vi "Address Claim.vi"(8 "error in (no error)":errorcluster, 11 "J1939 Main Configuration":T1={"Parameters"={"J1939 XNET Settings"={"XNET Database"="", "XNET Cluster"="", "CAN Port"="", "Baud rate [Bd]"=0, "Termination"=0, "Incoming Rate"=0, "Outcoming Rate"=1, "Write Decimation"=1}, "Incoming Single Point Configuraiton"={"Incoming Single Point Frame"={"ID"=[], "Conversion"=[], "Channel Array Positions"=[], "Frame Length"=[]}, "Channel Pairs"={"Chan Refs"=[], "Previous Chan Values"=[]}, "Read FIFO"=refnum}, "Outgoing Cyclic Configuraiton"={"Outgoing Cyclic Frame"={"ID"=[], "Conversion"=[], "Channel Array Positions"=[], "Frame Length"=[], "Transmit Propreties"=[]}, "Channel Pairs"={"Block Data Refs"=[], "Previous Chan Values"=[]}, "Write FIFO"=refnum}, "J1939 Monitor Settings"={"J1939 Network Address"=0, "Name"=0}, "Simulated Addresses"=[], "Simulated Addresses LUT"=variant}, "Name"="", "J1939 Cluster"={"Processed Incoming"=refnum, "Current Device Address"=0, "Processed Outgoing"=refnum, "Process Outgoing"=refnum, "Name"=0}, "References"={"BAM Buffer"=refnum, "CM Buffer"=refnum, "CM Gen"=refnum, "BAM Gen"=refnum, "Address Claims"=refnum, "RQST"=refnum}, "StopRef"=refnum, "Frame In"="", "Frame Out"="", "Incoming Timeout"=0, "Outgoing Timeout"=0, "Listener ID"=refnum, "Parent VI Ref"=refnum, "Data Ref"=refnum, "Scale Ref"=refnum, "Incoming Direct Access"={"Offset"=0, "Length"=0}, "Outgoing Direct Access"={"Offset"=0, "Length"=0}, "vi reference"=refnum, "Name and Address"="", "Simulated Addresses"=[], "Simulated Addresses LUT"=variant} {"Simulated Addresses"."Simulated Addresses"."J1939 XNET Settings"."Name" format="%.0x"; "Simulated Addresses"."Simulated Addresses"."DM1 Data"."Data Reference" format="%.0x"; "Simulated Addresses"."Simulated Addresses"."DM1 Enable?"."Data Reference" format="%.0x"; "Simulated Addresses"."Simulated Addresses"."DM2 Data"."Data Reference" format="%.0x"; "Simulated Addresses"."Simulated Addresses"."DM2 Enable?"."Data Reference" format="%.0x"; "Parameters"."Simulated Addresses"."Simulated Addresses"."J1939 XNET Settings"."Name" format="%.0x"; "Parameters"."J1939 Monitor Settings"."Name" format="%.0x"; "Parameters"."Outgoing Cyclic Configuraiton"."Channel Pairs"."Block Data Refs"."Data Reference" format="%.0x"; "Parameters"."Outgoing Cyclic Configuraiton"."Outgoing Cyclic Frame"."Transmit Propreties"."Transmit Time" format="%#_p"; "Parameters"."J1939 XNET Settings"."Termination" items=["Off", "On"]; "Parameters"."Incoming Single Point Configuraiton"."Channel Pairs"."Chan Refs" format="%.0x"}) -> (0 "error out":errorcluster, 3 "J1939 Main Configuration Out":T1={"Parameters"={"J1939 XNET Settings"={"XNET Database"="", "XNET Cluster"="", "CAN Port"="", "Baud rate [Bd]"=0, "Termination"=0, "Incoming Rate"=0, "Outcoming Rate"=1, "Write Decimation"=1}, "Incoming Single Point Configuraiton"={"Incoming Single Point Frame"={"ID"=[], "Conversion"=[], "Channel Array Positions"=[], "Frame Length"=[]}, "Channel Pairs"={"Chan Refs"=[], "Previous Chan Values"=[]}, "Read FIFO"=refnum}, "Outgoing Cyclic Configuraiton"={"Outgoing Cyclic Frame"={"ID"=[], "Conversion"=[], "Channel Array Positions"=[], "Frame Length"=[], "Transmit Propreties"=[]}, "Channel Pairs"={"Block Data Refs"=[], "Previous Chan Values"=[]}, "Write FIFO"=refnum}, "J1939 Monitor Settings"={"J1939 Network Address"=0, "Name"=0}, "Simulated Addresses"=[], "Simulated Addresses LUT"=variant}, "Name"="", "J1939 Cluster"={"Processed Incoming"=refnum, "Current Device Address"=0, "Processed Outgoing"=refnum, "Process Outgoing"=refnum, "Name"=0}, "References"={"BAM Buffer"=refnum, "CM Buffer"=refnum, "CM Gen"=refnum, "BAM Gen"=refnum, "Address Claims"=refnum, "RQST"=refnum}, "StopRef"=refnum, "Frame In"="", "Frame Out"="", "Incoming Timeout"=0, "Outgoing Timeout"=0, "Listener ID"=refnum, "Parent VI Ref"=refnum, "Data Ref"=refnum, "Scale Ref"=refnum, "Incoming Direct Access"={"Offset"=0, "Length"=0}, "Outgoing Direct Access"={"Offset"=0, "Length"=0}, "vi reference"=refnum, "Name and Address"="", "Simulated Addresses"=[], "Simulated Addresses LUT"=variant} {"Simulated Addresses"."Simulated Addresses"."J1939 XNET Settings"."Name" format="%.0x"; "Simulated Addresses"."Simulated Addresses"."DM1 Data"."Data Reference" format="%.0x"; "Simulated Addresses"."Simulated Addresses"."DM1 Enable?"."Data Reference" format="%.0x"; "Simulated Addresses"."Simulated Addresses"."DM2 Data"."Data Reference" format="%.0x"; "Simulated Addresses"."Simulated Addresses"."DM2 Enable?"."Data Reference" format="%.0x"; "Parameters"."Simulated Addresses"."Simulated Addresses"."J1939 XNET Settings"."Name" format="%.0x"; "Parameters"."J1939 Monitor Settings"."Name" format="%.0x"; "Parameters"."Outgoing Cyclic Configuraiton"."Channel Pairs"."Block Data Refs"."Data Reference" format="%.0x"; "Parameters"."Outgoing Cyclic Configuraiton"."Outgoing Cyclic Frame"."Transmit Propreties"."Transmit Time" format="%#_p"; "Parameters"."J1939 XNET Settings"."Termination" items=["Off", "On"]; "Parameters"."Incoming Single Point Configuraiton"."Channel Pairs"."Chan Refs" format="%.0x"})   [LabVIEW 2013, in "J1939 Addon Engine.lvlib"]
uses:
  Engine/J1939 Addon Engine.lvlib
  Engine/Types/Configuration Cluster.ctl
  Engine/Types/Process Parameters.ctl
  Types/XNET Settings.ctl
  Engine/Types/Incoming Single Point Configuration.ctl
  Engine/Types/Incoming Single Point Frame Pairs.ctl
  Engine/Types/Incoming Single Point Channel Pairs.ctl
  <vilib>/NI Veristand/Custom Device API/Data Reference.ctl
  Engine/Types/Outgoing Cyclic Configuration.ctl
  Engine/Types/Outgoing Cyclic Frame Pairs.ctl
  Types/XNET Frame Event Properties.ctl
  Engine/Types/Outgoing Cyclic Channel Pairs.ctl
  <vilib>/NI Veristand/Custom Device API/Block Data Reference.ctl
  Types/Monitor Settings.ctl
  Engine/Types/Simulated Settings.ctl
  Types/Compiled Simulated Settings.ctl
  Engine/Types/DTC FIFOs.ctl
  Types/Setup Information Cluster.ctl
  <vilib>/xnet/xnet.llb/XNET Frame CAN.ctl
  <vilib>/xnet/xnet.llb/XNET Frame Type CAN.ctl
  J1939 Utilities/Types/CAN Outgoing Message Cluster.ctl
  Types/TP List References.ctl
  Types/BAM Buffer Connections List_Ref.ctl
  Types/Connection Mode Generation Connection Ref.ctl
  Types/BAM Generation Connections List_Ref.ctl
  Types/Address Table Reference.ctl
  Types/RQST Lookup Table Reference.ctl
  Engine/SubVIs/Stop FG/Stop Global Ref.ctl
  Diagnostics Addon/Source/Engine/SubVIs/Datatable Lookup DVR.ctl
  Types/RQST Comm Lookup Table_Ref.ctl
  Types/Address Lookup Table Action.ctl
  J1939 Utilities/SubVIs/Convert CAN Data (U8) to U32.vi
  J1939 Utilities/SubVIs/Convert CAN Data (U32) to U8.vi
  J1939 Utilities/SubVIs/Convert CAN Arb ID to J1939 ID.vi
  J1939 Utilities/SubVIs/Convert J1939 ID to CAN Arb ID.vi
  <vilib>/xnet/xnet.llb/XNET Write (Frame CAN).vi
  J1939 Utilities/SubVIs/Request Address.vi
  <vilib>/xnet/xnet.llb/XNET Read.vi
  <vilib>/xnet/xnet.llb/XNET Read (Frame CAN).vi
  J1939 Utilities/J1939 Utilities.lvlib
  Engine/SubVIs/Error Handling API/Error Handling API.lvlib
  <vilib>/NI Veristand/Custom Device Tools/Custom Device Utility Library/Custom Device Utility Library.lvlib
  Engine/SubVIs/Stop FG/Stop FG.lvlib
  <vilib>/NI Veristand/Custom Device API/Custom Device API.lvlib
  J1939 Addon Shared.lvlib
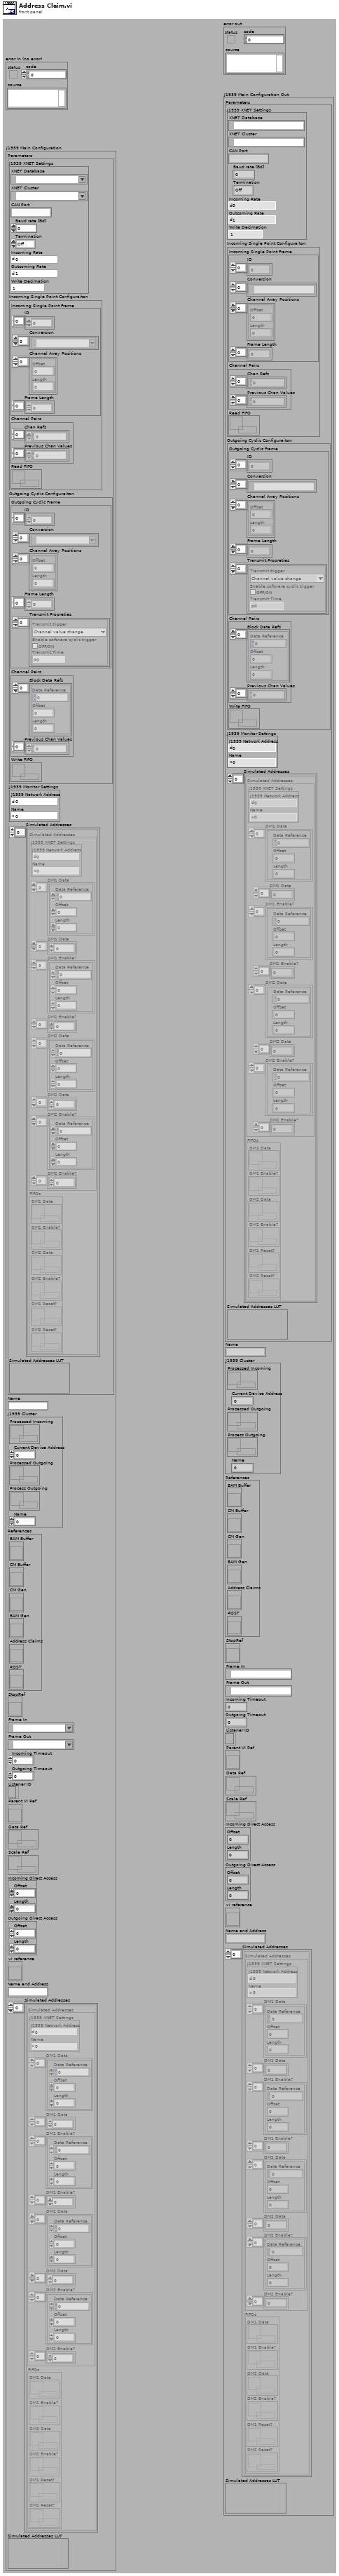
[diagram p1: front panel]
types:
  T1 = typedef "J1939 Addon Engine.lvlib/Configuration Cluster.ctl" = cluster{"Parameters":T2, "Name":string, "J1939 Cluster":T17, "References":T18, "StopRef":T24, "Frame In":refnum<k21>, "Frame Out":refnum<k21>, "Incoming Timeout":u32, "Outgoing Timeout":u32, "Listener ID":refnum<k5>, "Parent VI Ref":refnum<vi>, "Data Ref":refnum<data-value>, "Scale Ref":refnum<data-value>, "Incoming Direct Access":cluster{"Offset":u32, "Length":u32}, "Outgoing Direct Access":cluster{"Offset":u32, "Length":u32}, "vi reference":T25, "Name and Address":string, "Simulated Addresses":T14[], "Simulated Addresses LUT":variant}
  T2 = typedef "J1939 Addon Engine.lvlib/Process Parameters.ctl" = cluster{"J1939 XNET Settings":T3, "Incoming Single Point Configuraiton":T4, "Outgoing Cyclic Configuraiton":T8, "J1939 Monitor Settings":T13, "Simulated Addresses":T14[], "Simulated Addresses LUT":variant}
  T3 = typedef "J1939 Addon Shared.lvlib/XNET Settings.ctl" = cluster{"XNET Database":refnum<k21>, "XNET Cluster":refnum<k21>, "CAN Port":string, "Baud rate [Bd]":u32, "Termination":u32, "Incoming Rate":u32, "Outcoming Rate":u32, "Write Decimation":u32}
  T4 = typedef "J1939 Addon Engine.lvlib/Incoming Single Point Configuration.ctl" = cluster{"Incoming Single Point Frame":T5, "Channel Pairs":T6, "Read FIFO":refnum<k33>}
  T5 = typedef "J1939 Addon Engine.lvlib/Incoming Single Point Frame Pairs.ctl" = cluster{"ID":u32[], "Conversion":refnum<k21>[], "Channel Array Positions":cluster{"Offset":u32, "Length":u32}[], "Frame Length":u32[]}
  T6 = typedef "J1939 Addon Engine.lvlib/Incoming Single Point Channel Pairs.ctl" = cluster{"Chan Refs":T7[], "Previous Chan Values":dbl[]}
  T7 = typedef "Custom Device API.lvlib/Data Reference.ctl" = i32
  T8 = typedef "J1939 Addon Engine.lvlib/Outgoing Cyclic Configuration.ctl" = cluster{"Outgoing Cyclic Frame":T9, "Channel Pairs":T11, "Write FIFO":refnum<k33>}
  T9 = typedef "J1939 Addon Engine.lvlib/Outgoing Cyclic Frame Pairs.ctl" = cluster{"ID":u32[], "Conversion":refnum<k21>[], "Channel Array Positions":cluster{"Offset":u32, "Length":u32}[], "Frame Length":u32[], "Transmit Propreties":T10[]}
  T10 = typedef "J1939 Addon Shared.lvlib/XNET Frame Event Properties.ctl" = cluster{"Transmit trigger":enum16{"Channel value change"}, "Enable software cyclic trigger":bool, "Transmit Time":dbl}
  T11 = typedef "J1939 Addon Engine.lvlib/Outgoing Cyclic Channel Pairs.ctl" = cluster{"Block Data Refs":T12[], "Previous Chan Values":dbl[]}
  T12 = typedef "Custom Device API.lvlib/Block Data Reference.ctl" = cluster{"Data Reference":T7, "Offset":i32, "Length":i32}
  T13 = typedef "J1939 Addon Shared.lvlib/Monitor Settings.ctl" = cluster{"J1939 Network Address":u8, "Name":u64}
  T14 = typedef "J1939 Addon Engine.lvlib/Simulated Settings.ctl" = cluster{"Simulated Addresses":T15, "FIFOs":T16}
  T15 = typedef "J1939 Addon Shared.lvlib/Compiled Simulated Settings.ctl" = cluster{"J1939 XNET Settings":T13, "DM1 Data":T12[], "DM1 Data":dbl[], "DM1 Enable?":T12[], "DM1 Enable?":dbl[], "DM2 Data":T12[], "DM2 Data":dbl[], "DM2 Enable?":T12[], "DM2 Enable?":dbl[]}
  T16 = typedef "J1939 Addon Engine.lvlib/DTC FIFOs.ctl" = cluster{"DM1 Data":refnum<k33>, "DM1 Enable?":refnum<k33>, "DM2 Data":refnum<k33>, "DM2 Enable?":refnum<k33>, "DM1 Reset?":refnum<k33>, "DM2 Reset?":refnum<k33>}
  T17 = typedef "J1939 Addon Engine.lvlib/Setup Information Cluster.ctl" = cluster{"Processed Incoming":refnum<queue>, "Current Device Address":u8, "Processed Outgoing":refnum<queue>, "Process Outgoing":refnum<queue>, "Name":u64}
  T18 = typedef "J1939 Addon Engine.lvlib/TP List References.ctl" = cluster{"BAM Buffer":T19, "CM Buffer":T19, "CM Gen":T20, "BAM Gen":T21, "Address Claims":T22, "RQST":T23}
  T19 = typedef "J1939 Addon Engine.lvlib/BAM Buffer Connections List_Ref.ctl" = refnum<vi>
  T20 = typedef "J1939 Addon Engine.lvlib/Connection Mode Generation Connection Ref.ctl" = refnum<vi>
  T21 = typedef "J1939 Addon Engine.lvlib/BAM Generation Connections List_Ref.ctl" = refnum<vi>
  T22 = typedef "J1939 Addon Engine.lvlib/Address Table Reference.ctl" = refnum<vi>
  T23 = typedef "J1939 Addon Engine.lvlib/RQST Lookup Table Reference.ctl" = refnum<vi>
  T24 = typedef "J1939 Addon Engine.lvlib/Stop FG.lvlib/Stop Global Ref.ctl" = refnum<vi>
  T25 = typedef "J1939 Addon Engine.lvlib/RQST Comm Lookup Table_Ref.ctl" = refnum<vi>
  T26 = typedef "J1939 Addon Shared.lvlib/J1939 Utilities.lvlib/CAN Outgoing Message Cluster.ctl" = cluster{"Identifier":u32, "Data":u8[]}
  T27 = typedef "XNET Frame CAN.ctl" = cluster{"timestamp":timestamp, "payload":u8[], "identifier":u32, "type":T28, "extended?":bool, "echo?":bool}
  T28 = typedef "XNET Frame Type CAN.ctl" = u8
  T29 = typedef "J1939 Addon Shared.lvlib/J1939 Utilities.lvlib/Convert CAN Data (U8) Cluster.ctl" = cluster{"Byte 1":u8, "Byte 2":u8, "Byte 3":u8, "Byte 4":u8, "Byte 5":u8, "Byte 6":u8, "Byte 7":u8, "Byte 8":u8}
  T30 = typedef "J1939 Addon Engine.lvlib/Address Lookup Table Action.ctl" = enum16{"Initialize", "Add", "Get", "Remove", "Get All"}
  T31 = typedef "J1939 Addon Shared.lvlib/Address Lookup Table Data.ctl" = cluster{"Name":u8[], "Address":u8}
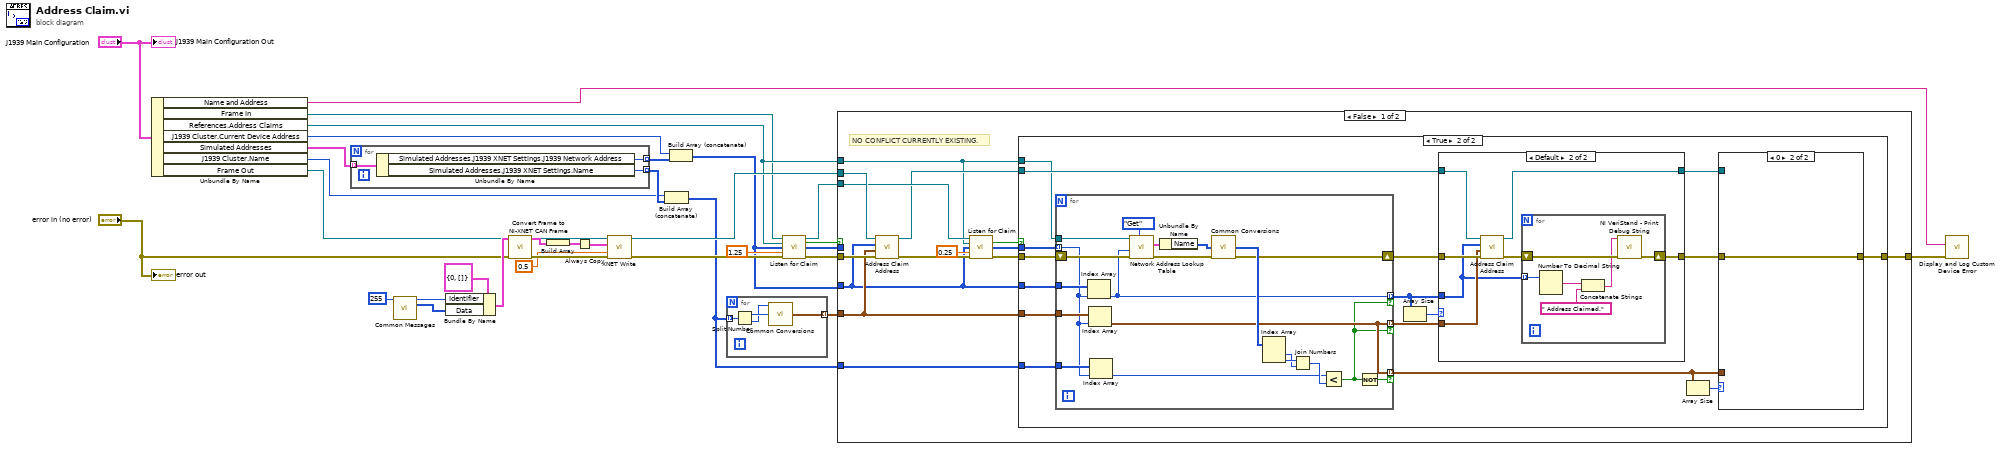
[diagram p0: block diagram]
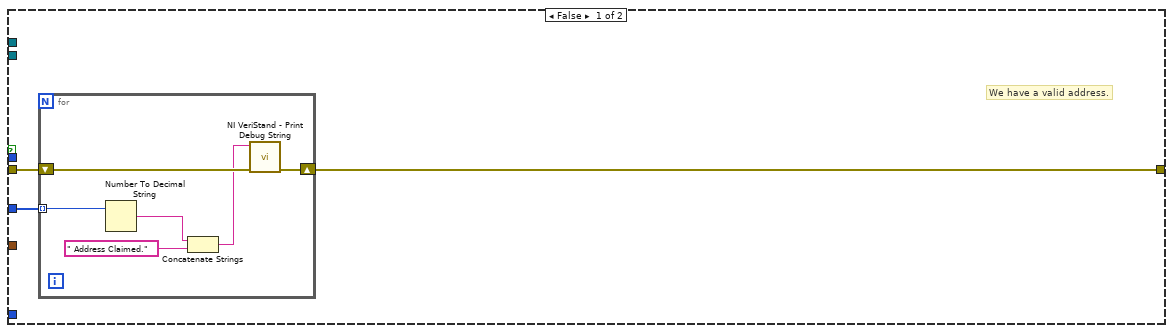
[diagram p2: hidden frame]
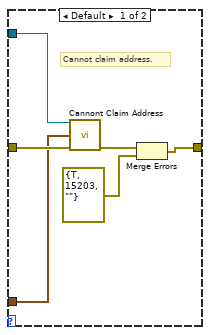
[diagram p3: hidden frame]
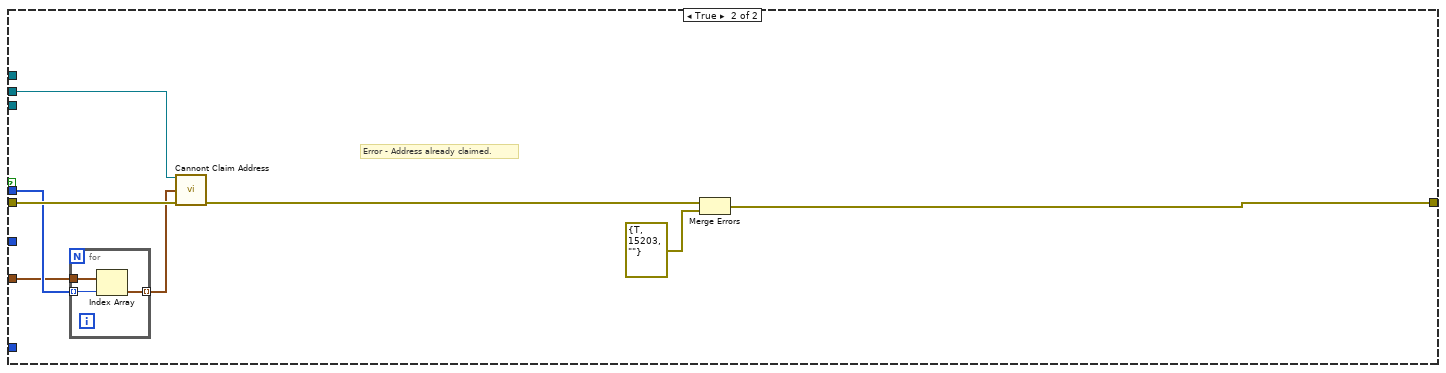
[diagram p5: hidden frame]
diagram:
  n1 = Unbundle By Name("J1939 Main Configuration") -> ("Name and Address"=w8:string, "Frame In"=w1:refnum<k21>, "References.Address Claims"=w13:T22, "J1939 Cluster.Current Device Address"=w12:u8, "Simulated Addresses"=w7:T14[], "J1939 Cluster.Name"=w4:u64, "Frame Out"=w2:refnum<k21>)
  n2 = for {
    tunnel: w7 -> [w35] mode=indexing
    tunnel: [w33] -> w6 mode=indexing
    tunnel: [w34] -> w5 mode=indexing
    n3 = Unbundle By Name(w35) -> ("Simulated Addresses.J1939 XNET Settings.J1939 Network Address"=w33:u8, "Simulated Addresses.J1939 XNET Settings.Name"=w34:u64)
  }
  n4 = call-poly "Common Messages.vi"("Destination Address"=u8 255) -> ("Arb ID"=w32:u32, "Data"=w31:u8[])  [unwired: 13 in]
  n5 = Bundle By Name(cluster=T26 {"Identifier"=0, "Data"=[]} ("Data to Send"), "Identifier"=w32, "Data"=w31) -> (w29:T26)
  n6 = call "Convert Frame to NI-XNET CAN Frame.vi"("error in (no error)"="error in (no error)", "Data to Send"=w29) -> ("error out"=w27:errorcluster, "CAN frame"=w28:T27)  [unwired: 8 in]
  n7 = Build Array(w28) -> (w17:T27[])
  n8 = Always Copy(1:w17) -> (0:w11:T27[])
  n9 = call-poly <vilib>:"XNET Write.vi"("session in"=w2, "data"=w11, "timeout (10)"=0.5, "error in (no error)"=w27) -> ("session out"=w21:refnum<k21>, "error out"=w26:errorcluster)  [unwired: 10 out]
  n10 = Build Array (concatenate)(w4, w5) -> (w10:u64[])
  n11 = Build Array (concatenate)(w12, w6) -> (w3:u8[])
  n12 = for {
    tunnel: [w36] -> w20 mode=indexing
    tunnel: w10 -> [w37] mode=indexing
    n13 = Split Number(x=w37) -> (hi(x)=w39:u32, lo(x)=w38:u32)
    n14 = call-poly "Common Conversions.vi"("Data 0-3"=w38, "Data 4-7"=w39) -> ("Byte Cluster"=w36:T29)  [unwired: 13 in]
  }
  n15 = call "Listen for Claim.vi"("session in"=w1, "ref in"=w13, "Requested Addresses"=w3, "timeout (0)"=1.25, "error in"=w26) -> ("session out"=w23:refnum<k21>, "Conflict?"=w24:bool, "Conflict Indeces"=w9:i32[], "error out"=w22:errorcluster)  [unwired: 7 in]
  n16 = case shown="False" w24 {
    tunnel: w3 -> [w41 _]
    tunnel: w10 -> [w48 _]
    tunnel: w23 -> [w50 _]
    tunnel: w22 -> [w51 w127]
    tunnel: w21 -> [w52 w126]
    tunnel: [w44 w123] -> w16
    tunnel: w20 -> [w43 w121]
    tunnel: w13 -> [w42 _]
    tunnel: w9 -> [_ w122]
    frame False {
      # "NO CONFLICT CURRENTLY EXISTING."
      n17 = call "Address Claim Address.vi"("error in"=w51, "Names"=w43, "Requested Addresses"=w41, "session in"=w52) -> ("error out"=w53:errorcluster, "session out"=w46:refnum<k21>)  [unwired: 6 in]
      n18 = call "Listen for Claim.vi"("session in"=w50, "ref in"=w42, "Requested Addresses"=w41, "timeout (0)"=0.25, "error in"=w53) -> ("Conflict?"=w47:bool, "Conflict Indeces"=w40:i32[], "error out"=w45:errorcluster)  [unwired: 7 in, 1 out]
      n19 = case shown="True" w47 {
        tunnel: w48 -> [_ w70]
        tunnel: w46 -> [_ w78]
        tunnel: w45 -> [w56 w77]
        tunnel: w43 -> [_ w72]
        tunnel: [w55 w65] -> w44
        tunnel: w42 -> [_ w75]
        tunnel: w41 -> [w54 w71]
        tunnel: w40 -> [_ w74]
        frame False {
          # "We have a valid address."
          n20 = for {
            shift-right: [w61] -> w55
            shift-left: w56 -> [w62]
            tunnel: w54 -> [w58] mode=indexing
            n21 = Number To Decimal String(number=w58) -> (decimal integer string=w57:string)  [unwired: 1 in]
            n22 = Concatenate Strings(w57, " Address Claimed." ("string")) -> (w59:string)
            n23 = call <vilib>:"NI VeriStand - Print Debug String.vi"("error in (no error)"=w62, "Message"=w59) -> ("error out"=w61:errorcluster)  [unwired: 9 in]
          }
        }
        frame True {
          n24 = for {
            tunnel: w75 -> [w97]
            tunnel: w74 -> [w88] mode=indexing
            tunnel: [w90] -> w73 mode=indexing if=w87
            tunnel: w72 -> [w94]
            tunnel: w71 -> [w93]
            tunnel: [w86] -> w69 mode=indexing if=w87
            tunnel: w70 -> [w92]
            shift-right: [w98] -> w76
            shift-left: w77 -> [w99]
            tunnel: [w90] -> w63 mode=indexing if=w89
            n25 = Index Array(array=w93, index=w88) -> (element=w86:u8)
            n26 = Index Array(array=w94, index=w88) -> (element=w90:T29)
            n27 = Index Array(array=w92, index=w88) -> (element=w91:u64)
            n28 = call "Network Address Lookup Table.vi"("Action"=Address_Lookup_Table_Action."Get", "error in (no error)"=w99, "Address"=w86, "ref in"=w97) -> ("error out"=w98:errorcluster, "Data"=w96:T31)  [unwired: 4 in, 2 out]
            n29 = Unbundle By Name(w96) -> ("Name"=w95:u8[])
            n30 = call-poly "Common Conversions.vi"("Data"=w95) -> ("Array"=w104:u32[])  [unwired: 14 in]
            n31 = Index Array(array=w104) -> (element #1=w102:u32, element #2=w103:u32)  [unwired: 2 in]
            n32 = Join Numbers(hi=w103, lo=w102) -> ((hi.lo)=w101:u64)
            n33 = Less?(x=w91, y=w101) -> (x < y?=w87:bool)
            n34 = Not(x=w87) -> (.not. x?=w89:bool)
          }
          n35 = Array Size(array=w69) -> (size(s)=w68:i32)
          n36 = case shown="Default" w68 {
            tunnel: w78 -> [w105 w112]
            tunnel: w76 -> [w106 w113]
            tunnel: w73 -> [_ w111]
            tunnel: [w106 w109] -> w66
            tunnel: w69 -> [_ w107]
            tunnel: [w105 w108] -> w67
            frame 0 {
            }
            frame Default {
              n37 = call "Address Claim Address.vi"("error in"=w113, "Names"=w111, "Requested Addresses"=w107, "session in"=w112) -> ("error out"=w110:errorcluster, "session out"=w108:refnum<k21>)  [unwired: 6 in]
              n38 = for {
                shift-right: [w118] -> w109
                shift-left: w110 -> [w119]
                tunnel: w107 -> [w117] mode=indexing
                n39 = Number To Decimal String(number=w117) -> (decimal integer string=w116:string)  [unwired: 1 in]
                n40 = Concatenate Strings(w116, " Address Claimed." ("string")) -> (w115:string)
                n41 = call <vilib>:"NI VeriStand - Print Debug String.vi"("error in (no error)"=w119, "Message"=w115) -> ("error out"=w118:errorcluster)  [unwired: 9 in]
              }
            }
          }
          n42 = Array Size(array=w63) -> (size(s)=w64:i32)
          n43 = case shown="0" w64 {
            tunnel: w67 -> [w82 _]
            tunnel: w66 -> [w84 w85]
            tunnel: w63 -> [w83 _]
            tunnel: [w79 w85] -> w65
            frame Default {
              # "Cannot claim address."
              n44 = call "Cannont Claim Address.vi"("session out"=w82, "Names"=w83, "error in"=w84) -> ("error out"=w81:errorcluster)  [unwired: 12 in]
              n45 = Merge Errors(w81, errorcluster {"status"=TRUE, "code"=15203, "source"=""} ("error out")) -> (w79:errorcluster)
            }
            frame 0 {
            }
          }
        }
      }
    }
    frame True {
      # "Error - Address already claimed."
      n46 = for {
        tunnel: w122 -> [w129] mode=indexing
        tunnel: w121 -> [w130]
        tunnel: [w128] -> w120 mode=indexing
        n47 = Index Array(array=w130, index=w129) -> (element=w128:T29)
      }
      n48 = call "Cannont Claim Address.vi"("session out"=w126, "Names"=w120, "error in"=w127) -> ("error out"=w124:errorcluster)  [unwired: 12 in]
      n49 = Merge Errors(w124, errorcluster {"status"=TRUE, "code"=15203, "source"=""} ("error out")) -> (w123:errorcluster)
    }
  }
  n50 = call "Display and Log Custom Device Error.vi"("error out"=w16, "Your code's public name"=w8) -> ()  [unwired: 10 in]
  "error out" <- "error in (no error)"
  "J1939 Main Configuration Out" <- "J1939 Main Configuration"
